vi "Do Selection.vi"(8 "error in":errorcluster, 10 "IPopulation in":refnum<class "IPopulation.lvclass">, 11 "Selector in":refnum<class "Selector.lvclass">) -> (0 "error out":errorcluster, 2 "IPopulation out":refnum<class "IPopulation.lvclass">, 3 "Selector out":refnum<class "Selector.lvclass">)   [LabVIEW 2016, in "Selector.lvclass"]
uses:
  Selector.lvclass
  IPopulation/IPopulation.lvclass
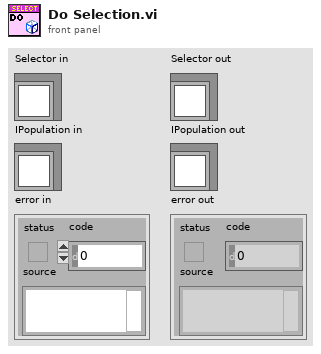
[diagram p1: front panel]
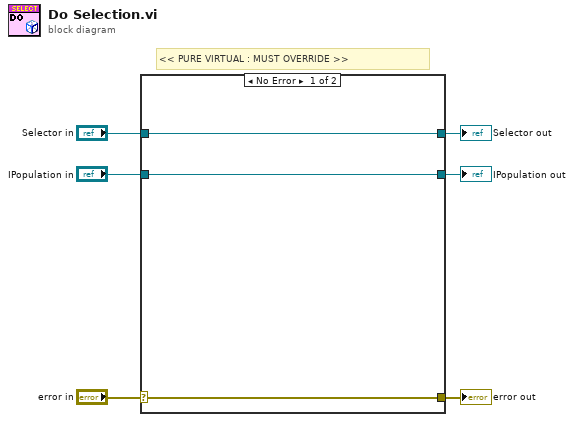
[diagram p0: block diagram]
diagram:
  # "<< PURE VIRTUAL : MUST OVERRIDE >>"
  n1 = case shown="No Error" "error in" {
    selector: "error in" -> [w8 w12]
    tunnel: [w8 w12] -> w5
    tunnel: [w9 w11] -> w3
    tunnel: "Selector in" -> [w9 w11]
    tunnel: "IPopulation in" -> [w7 w10]
    tunnel: [w7 w10] -> w1
    frame No Error {
    }
    frame Error {
    }
  }
  "error out" <- w5
  "Selector out" <- w3
  "IPopulation out" <- w1
